vi "OP500ZP_OuCrash.vi"(2 "Booléen":bool, 3 "in":T1=enum."Scan") -> (0 "OUT":T1=enum."Scan")   [LabVIEW 2020]
uses:
  OP500ZP_state.ctl
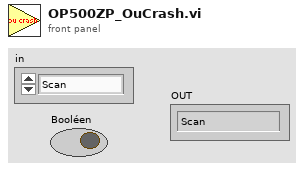
[diagram p1: front panel]
types:
  T1 = typedef "OP500ZP_state.ctl" = enum16{"Null", "Demarrage", "Init", "Scan", "Iso", "Softs", "MCU", "OCVACIR", "Conti", "DTC", "DataDyn", "DataDyn2", "Crash", "Next", "Comext"}
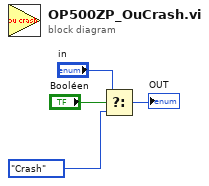
[diagram p0: block diagram]
diagram:
  n1 = Select(t="in", s="Booléen", f=OP500ZP_state."Crash") -> (s? t:f=→"OUT":T1)
